vi "perform_measurement.vi"(7 "DAQmx Device Name":tag="Dev1", 8 "error in":errorcluster, 11 "Stimuli":T2) -> (0 "error out":errorcluster, 2 "Load Set":T1, 3 "Outputs":T4)   [LabVIEW 2024]
doc: "The VI performs a measurement with the exctication defined in Stimuli cluster. \n- Based on the Stimuli input cluster the measurement environment cluster is generated by get_meas_env.vi\n- At first the resistive loads are set (set_loads.vi). The Load Set is provided also as output indicator\n- After 200 ms waiting the test outputs are generated (get_test_output.vi). The outpu is ctl_test_outputs_cluster"
uses:
  ctl_test_outputs_cluster.ctl
  ctl_stimuli_cluster.ctl
  ctl_loads_enum.ctl
  ctl_load_set_cluster.ctl
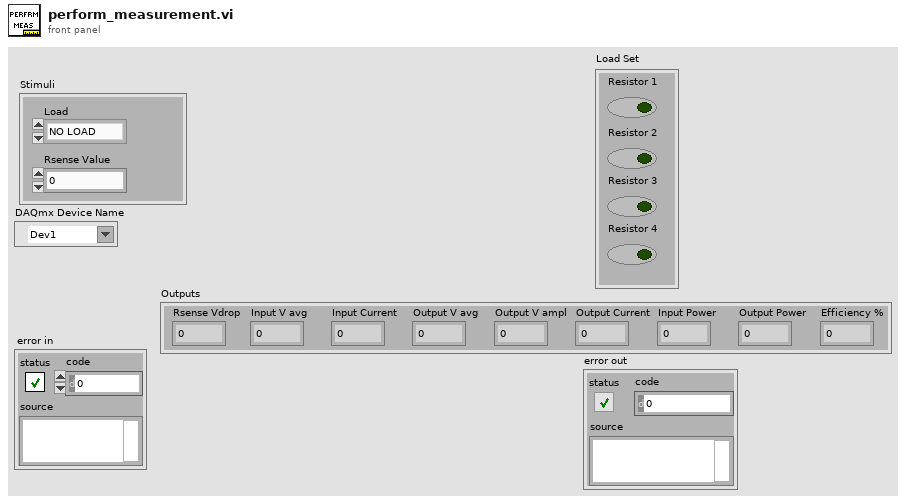
[diagram p1: front panel]
types:
  T1 = typedef "ctl_load_set_cluster.ctl" = cluster{"Resistor 1":bool, "Resistor 2":bool, "Resistor 3":bool, "Resistor 4":bool}
  T2 = typedef "ctl_stimuli_cluster.ctl" = cluster{"Load":T3, "Rsense Value":dbl}
  T3 = typedef "ctl_loads_enum.ctl" = enum16{"NO LOAD", "10Ohm", "6.8Ohm", "4.7Ohm", "3.3Ohm", "2.4Ohm", "1.6Ohm", "1.3Ohm"}
  T4 = typedef "ctl_test_outputs_cluster.ctl" = cluster{"Output V avg":dbl, "Output V ampl":dbl, "Input Current":dbl, "Output Current":dbl, "Efficiency %":dbl, "Input V avg":dbl, "Input Power":dbl, "Output Power":dbl, "Rsense Vdrop":dbl}
  T5 = typedef "ctl_meas_env_cluster.ctl" = cluster{"Rsense_value Ohm":dbl, "Rload_value Ohm":dbl}
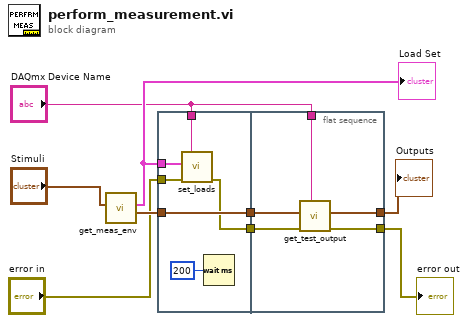
[diagram p0: block diagram]
diagram:
  n1 = call "get_meas_env.vi"("Stimuli"="Stimuli") -> ("Meas environment"=w7:T5, "Load Set"=w6:T1)  [unwired: 9 in]
  "Load Set" <- w6
  n2 = flat-sequence {
    tunnel: w6 -> [w15]
    tunnel: w7 -> [w14]
    tunnel: [w14] -> w9
    tunnel: [w12] -> w4
    tunnel: "error in" -> [w11]
    tunnel: "DAQmx Device Name" -> [w10]
    tunnel: w9 -> [w20]
    tunnel: [w19] -> w8
    tunnel: w4 -> [w18]
    tunnel: [w17] -> w3
    tunnel: "DAQmx Device Name" -> [w16]
    frame #0 {
      n3 = call "set_loads.vi"("DAQmx Device Name"=w10, "error in"=w11, "Load Set"=w15) -> ("error out"=w12:errorcluster)  [unwired: 8 in]
      n4 = Wait (ms)(milliseconds to wait=u32 200) -> ()  [unwired: 1 out]
    }
    frame #1 {
      n5 = call "get_test_output.vi"("DAQmx Device Name"=w16, "error in"=w18, "Meas environment"=w20) -> ("error out"=w17:errorcluster, "Outputs"=w19:T4)  [unwired: 7 in]
    }
  }
  "Outputs" <- w8
  "error out" <- w3
